vi "Update Corners.vi"() -> ()   [LabVIEW 2009]
uses:
  <vilib>/Analysis/Matrix/Datatypes/RealMatrix.ctl
  <vilib>/Analysis/Matrix/NI_Matrix.lvlib
panel:
  out "New Corners":cluster{"X":dbl, "Y":dbl}[](array[cluster])
  in  "Old corners":cluster{"X":dbl, "Y":dbl}[](array[cluster])
  in  "Added Points":cluster{"X":dbl, "Y":dbl}[](array[cluster])
  in  "Updated Map":T1
  in  "# safety grids":i32=4
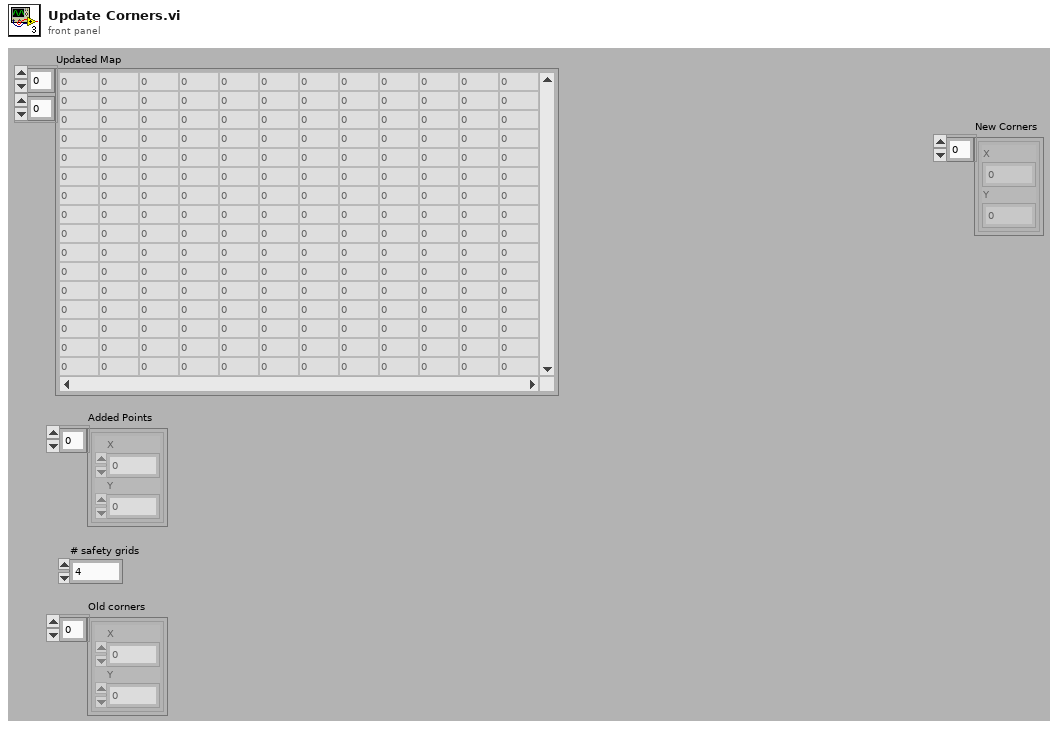
[diagram p1: front panel]
types:
  T1 = typedef "NI_Matrix.lvlib/RealMatrix.ctl" = dbl[][]
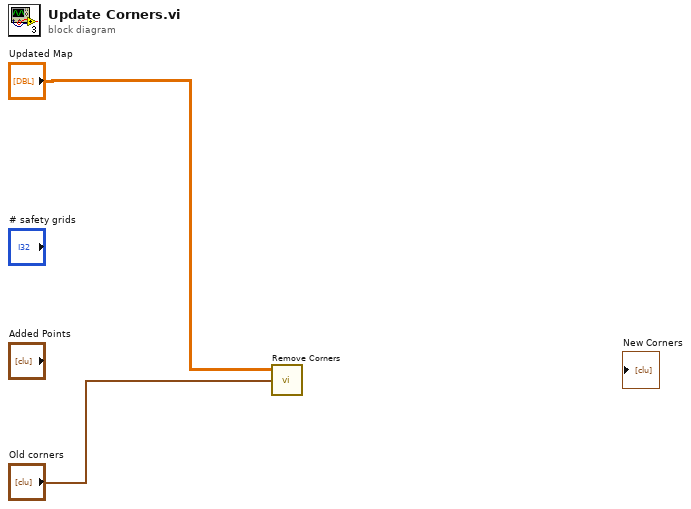
[diagram p0: block diagram]
diagram:
  n1 = call "Remove Corners.vi"("Old corners"="Old corners", "Updated Map"="Updated Map") -> ()  [unwired: 2 in, 1 out]
